vi "GetCameraConfiguration.vi"(8 "error in (no error)":errorcluster, 10 "camera":T1) -> (0 "error out":errorcluster, 1 "camera settings":T5={"emissitivity"=0.99, "reflected temperature"=273.15, "window transmission"=0.99, "window temperature"=273.15, "atmospheric transmission"=0.99, "atmospheric temperature"=273.15}, 3 "units":string="C")   [LabVIEW 2017, in "IrAcquisition.lvlib"]
uses:
  <vilib>/addons/InsightCM/Devices/Shared/Ir/IrAcquisition/IrAcquisition.lvlib
  <vilib>/addons/InsightCM/Devices/Shared/Ir/IrAcquisition/controls/IRCameraSettings.ctl
  <vilib>/addons/InsightCM/MessageBus/Base/controls/Camera.ctl
  <vilib>/addons/InsightCM/MessageBus/Base/controls/KeyValuePair.ctl
  <vilib>/addons/InsightCM/MessageBus/Base/controls/Trigger.ctl
  <vilib>/addons/InsightCM/MessageBus/Base/controls/Condition.ctl
  <vilib>/addons/InsightCM/Utilities/PropertyHelpers/PropertyHelpers.lvlib
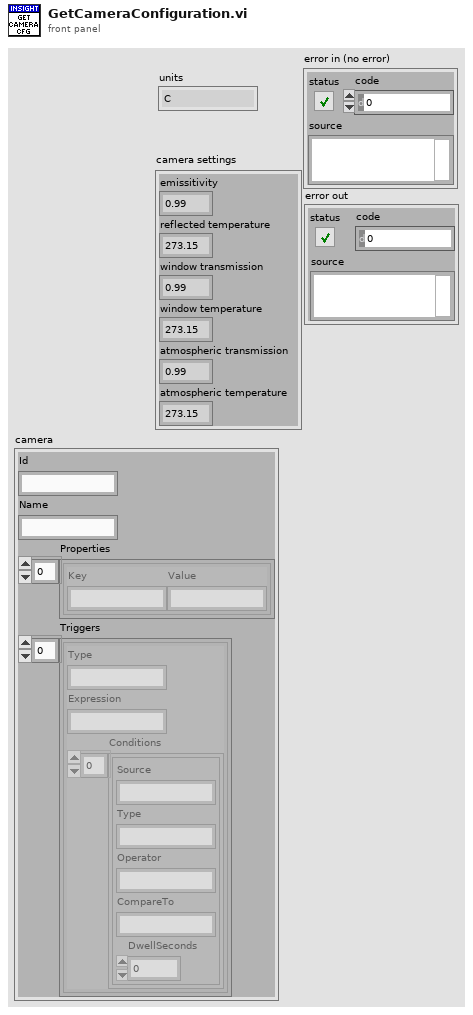
[diagram p1: front panel]
types:
  T1 = typedef "Camera.ctl" = cluster{"Id":string, "Name":string, "Properties":T2[], "Triggers":T3[]}
  T2 = typedef "KeyValuePair.ctl" = cluster{"Key":string, "Value":string}
  T3 = typedef "Trigger.ctl" = cluster{"Type":string, "Expression":string, "Conditions":T4[]}
  T4 = typedef "Condition.ctl" = cluster{"Source":string, "Type":string, "Operator":string, "CompareTo":string, "DwellSeconds":dbl}
  T5 = typedef "IrAcquisition.lvlib/IRCameraSettings.ctl" = cluster{"emissitivity":dbl, "reflected temperature":dbl, "window transmission":dbl, "window temperature":dbl, "atmospheric transmission":dbl, "atmospheric temperature":dbl}
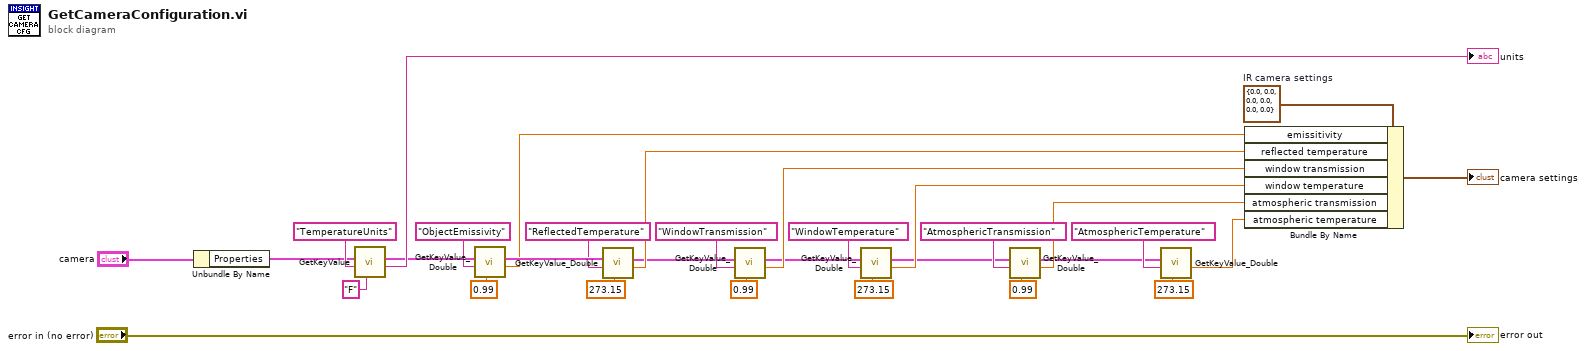
[diagram p0: block diagram]
diagram:
  w26 = T5 {"emissitivity"=0.0, "reflected temperature"=0.0, "window transmission"=0.0, "window temperature"=0.0, "atmospheric transmission"=0.0, "atmospheric temperature"=0.0}  # IR camera settings
  n1 = Unbundle By Name("camera") -> ("Properties"=w2:T2[])
  n2 = call <vilib>:"GetKeyValue.vi"("default value"="F", "key"="TemperatureUnits", "key value pairs"=w2) -> ("value"=→"units":string, "key value pairs out"=w1:T2[])  [unwired: 6 in, 1 out]
  n3 = call <vilib>:"GetKeyValue_Double.vi"("default"=0.99, "key"="ObjectEmissivity", "key value pairs"=w1) -> ("value"=w22:dbl, "key value pairs out"=w24:T2[])  [unwired: 6 in, 1 out]
  n4 = call <vilib>:"GetKeyValue_Double.vi"("default"=273.15, "key"="ReflectedTemperature", "key value pairs"=w24) -> ("value"=w21:dbl, "key value pairs out"=w18:T2[])  [unwired: 6 in, 1 out]
  n5 = call <vilib>:"GetKeyValue_Double.vi"("default"=0.99, "key"="WindowTransmission", "key value pairs"=w18) -> ("value"=w17:dbl, "key value pairs out"=w14:T2[])  [unwired: 6 in, 1 out]
  n6 = call <vilib>:"GetKeyValue_Double.vi"("default"=273.15, "key"="WindowTemperature", "key value pairs"=w14) -> ("value"=w13:dbl, "key value pairs out"=w10:T2[])  [unwired: 6 in, 1 out]
  n7 = call <vilib>:"GetKeyValue_Double.vi"("default"=0.99, "key"="AtmosphericTransmission", "key value pairs"=w10) -> ("value"=w9:dbl, "key value pairs out"=w6:T2[])  [unwired: 6 in, 1 out]
  n8 = call <vilib>:"GetKeyValue_Double.vi"("default"=273.15, "key"="AtmosphericTemperature", "key value pairs"=w6) -> ("value"=w5:dbl)  [unwired: 6 in, 2 out]
  n9 = Bundle By Name(cluster=w26, "emissitivity"=w22, "reflected temperature"=w21, "window transmission"=w17, "window temperature"=w13, "atmospheric transmission"=w9, "atmospheric temperature"=w5) -> (→"camera settings":T5)
  "error out" <- "error in (no error)"
